vi "Autonomous Independent.vi"   [LabVIEW 2014]
doc: "This VI is called when autonomous begins, and will automatically be terminated when autonomous ends. You can carry out timed or sensor driven robot movement independently without needing to return to the caller."
uses:
  <vilib>/Rock Robotics/WPI/Joystick/WPI_JoystickGetSetRefNum.vi
  <vilib>/Rock Robotics/Network Tables/SD Write Numeric Array.vi
  Robot Global Data.vi
  <vilib>/Rock Robotics/WPI/RobotDrive/WPI_RobotDriveGetSetRefNum.vi
types:
  T1 = typedef "WPI_JoystickDevRef.ctl" = cluster{"Device":T2}
  T2 = typedef "WPI_JoystickDeviceEnum.ctl" = enum16{"USB 0", "USB 1", "USB 2", "USB 3", "USB 4", "USB 5"}
  T3 = typedef "WPI_RobotDriveDevRef.ctl" = cluster{"DevStatus":errorcluster, "Motors[]":T4[], "Square Inputs":bool, "Max Output":dbl}
  T4 = typedef "WPI_MotorControlDeviceRef.ctl" = cluster{"DeviceStatus":errorcluster, "Type":T5, "PWM":cluster{"Controller":T6, "PWM Channel":T7, "DeadBand":T8}, "CAN":cluster{"Device Number":u8, "Control Mode":T9, "Semaphore":T10, "Max Vout":dbl, "TalonSRX Control Mode":T11}, "Invert":bool, "TransformRef":T12, "InvTransformRef":T12}
  T5 = typedef "WPI_MotorControlType.ctl" = enum16{"PWM", "CAN", "CANTalonSRX"}
  T6 = typedef "FPGA_TypedefDigitalModule.ctl" = enum16{"Controller 1"}
  T7 = typedef "FPGA_DIOPWMChannel.ctl" = enum8{"PWM 0", "PWM 1", "PWM 2", "PWM 3", "PWM 4", "PWM 5", "PWM 6", "PWM 7", "PWM 8", "PWM 9", "PWM MXP 0", "PWM MXP 1", "PWM MXP 2", "PWM MXP 3", "PWM MXP 4", "PWM MXP 5", "PWM MXP 6", "PWM MXP 7", "PWM MXP 8", "PWM MXP 9", "Invalid"}
  T8 = typedef "WPI_PWMDeadband.ctl" = cluster{"Name":string, "maxPositivePwm":i32, "minPositivePwm":i32, "centerPwm":i32, "maxNegativePwm":i32, "minNegativePwm":i32, "angularRange":u16}
  T9 = typedef "WPI_CANJaguar_ControlMode.ctl" = enum8{"Percent VBus", "Current", "Speed", "Position", "Voltage"}
  T10 = typedef "Semaphore RefNum" = refnum<k1>
  T11 = typedef "WPI_CANTalonSRX_APIControlMode.ctl" = enum8{"Percent VBus", "Speed", "Position", "Slave", "Unchanged / Invalid"}
  T12 = typedef "WPI_PWMTransform_ConPane.ctl" = refnum<vi>
  T13 = typedef "WPI_CANTalonSRX_GlobalStatus.ctl" = cluster{"Applied Throttle":dbl, "Module Enabled":bool, "CAN Error":errorcluster, "Closed Loop Error":dbl, "Forward Limit Switch Closed":bool, "Reverse Limit Switch Closed":bool, "Sensor Position":dbl, "Sensor Velocity":dbl, "Current":dbl, "Sticky Fault - Over Temp":bool, "Sticky Fault - Under Voltage":bool, "Sticky Fault - Forward Limit":bool, "Sticky Fault - Reverse Limit":bool, "Sticky Fault - Forward Soft Limit":bool, "Sticky Fault - Reverse Soft Limit":bool, "Brake is Enabled":bool, "Encoder Position":dbl, "Encoder Velocity":dbl, "Encoder Index Count":dbl, "Encoder A Pin State":bool, "Encoder B Pin State":bool, "Encoder Index Pin State":bool, "Analog In":dbl, "Analog In Velocity":dbl, "Temperature (C)":dbl, "Battery Voltage":dbl}
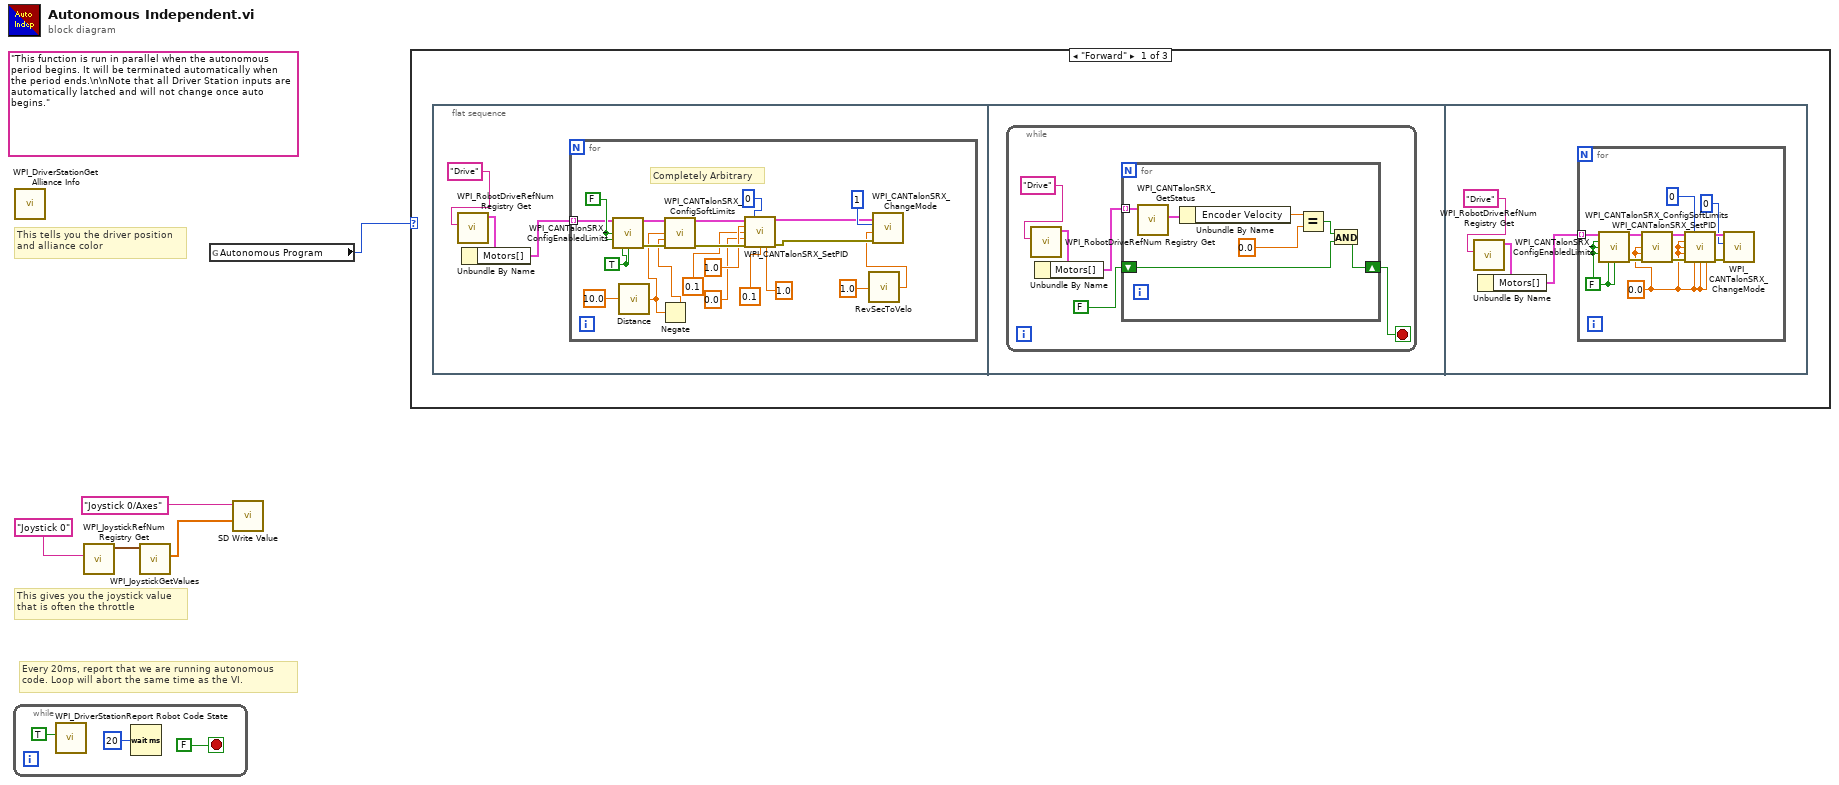
[diagram p0: block diagram]
diagram:
  (unwired) "This function is run in parallel when the autonomous period begins. It will be terminated automatically when the period ends.\n\nNote that all Driver Station inputs are automatically latched and will not change once auto begins."
  # "Every 20ms, report that we are running autonomous\ncode. Loop will abort the same time as the VI."
  # "This gives you the joystick value\nthat is often the throttle"
  # "This tells you the driver position\nand alliance color"
  n1 = while {
    stop <- FALSE stop-if-true
    n2 = call <vilib>:"WPI_DriverStationReport Robot Code State.vi"("Autonomous"=TRUE) -> ()  [unwired: 10 in, 1 out]
    n3 = Wait (ms)(milliseconds to wait=u32 20) -> ()  [unwired: 1 out]
  }
  n4 = call <vilib>:"WPI_DriverStationGet Alliance Info.vi"() -> ()  [unwired: 12 out]
  n5 = call <vilib>:"WPI_JoystickRefNum Registry Get.vi"("refnum name"="Joystick 0") -> ("JoystickDevRef"=w4:T1)  [unwired: 1 in, 9 out]
  n6 = call <vilib>:"WPI_JoystickGetValues.vi"("JoystickDevRef"=w4) -> ("Axes"=w2:dbl[])  [unwired: 6 in, 4 out]
  n7 = global read "Robot Global Data.vi" "Autonomous Program"() -> (w1:enum16{"Forward", "Stack", "Null"})
  n8 = call-poly <vilib>:"SD Write Value.vi"("Numeric Array"=w2, "Name"="Joystick 0/Axes") -> ()  [unwired: 8 in, 2 out]
  n9 = case shown="\"Forward\"" w1 {
    frame "Forward" {
      n10 = flat-sequence {
        frame #0 {
          n11 = call <vilib>:"WPI_RobotDriveRefNum Registry Get.vi"("refnum name"="Drive") -> ("RobotDriveDevRef"=w11:T3)  [unwired: 9 in, 1 out]
          n12 = Unbundle By Name(w11) -> ("Motors[]"=w9:T4[])
          n13 = for {
            tunnel: w9 -> [w17] mode=indexing
            w31 = TRUE
            w32 = FALSE
            # "Completely Arbitrary"
            n14 = call <vilib>:"WPI_CANTalonSRX_ConfigEnabledLimits.vi"("CAN Talon SRX Ref"=w17, "Forward Limit Switch Enable"=w32, "Reverse Limit Switch Enable"=w32, "Forward Soft Limit Enable"=w31, "Reverse Soft Limit Enable"=w31) -> ("CAN Talon SRX Ref Out"=w30:T4, "error out"=w29:errorcluster)  [unwired: 9 in]
            n15 = call "Distance.vi"("Revolutions"=10.0) -> ("Distance"=w13:dbl)
            n16 = Negate(x=w13) -> (-x=w12:dbl)
            n17 = call <vilib>:"WPI_CANTalonSRX_ConfigSoftLimits.vi"("CAN Talon SRX Ref"=w30, "Forward Limit Position"=w13, "Reverse Limit Position"=w12, "error in (no error)"=w29) -> ("CAN Talon SRX Ref Out"=w27:T4, "error out"=w26:errorcluster)  [unwired: 10 in]
            n18 = call <vilib>:"WPI_CANTalonSRX_SetPID.vi"("CAN Talon SRX Ref"=w27, "Parameter Slot"=0, "P"=1.0, "I"=0.1, "D"=0.0, "error in (no error)"=w26, "I Zone"=0.1, "Ramp Rate"=1.0) -> ("CAN Talon SRX Ref Out"=w24:T4, "error out"=w25:errorcluster)  [unwired: 6 in]
            n19 = call "RevSecToVelo.vi"("Revolutions/s"=1.0) -> ("Velocity"=w15:dbl)
            n20 = call <vilib>:"WPI_CANTalonSRX_ChangeMode.vi"("error in (no error)"=w25, "Output"=w15, "Control Mode"=1, "CAN Talon SRX Ref"=w24) -> ()  [unwired: 6 in, 2 out]
          }
        }
        frame #1 {
          n21 = while {
            stop <- w33 stop-if-true
            n22 = call <vilib>:"WPI_RobotDriveRefNum Registry Get.vi"("refnum name"="Drive") -> ("RobotDriveDevRef"=w36:T3)  [unwired: 9 in, 1 out]
            n23 = Unbundle By Name(w36) -> ("Motors[]"=w35:T4[])
            n24 = for {
              tunnel: w35 -> [w41] mode=indexing
              shift-right: [w39] -> w33
              shift-left: FALSE -> [w38]
              n25 = call <vilib>:"WPI_CANTalonSRX_GetStatus.vi"("CAN Talon SRX Ref"=w41) -> ("Talon SRX Status"=w44:T13)  [unwired: 8 in, 2 out]
              n26 = Unbundle By Name(w44) -> ("Encoder Velocity"=w43:dbl)
              n27 = Equal?(x=w43, y=0.0) -> (x = y?=w40:bool)
              n28 = And(x=w40, y=w38) -> (x .and. y?=w39:bool)
            }
          }
        }
        frame #2 {
          n29 = call <vilib>:"WPI_RobotDriveRefNum Registry Get.vi"("refnum name"="Drive") -> ("RobotDriveDevRef"=w46:T3)  [unwired: 9 in, 1 out]
          n30 = Unbundle By Name(w46) -> ("Motors[]"=w45:T4[])
          n31 = for {
            tunnel: w45 -> [w58] mode=indexing
            w51 = 0.0
            w57 = FALSE
            n32 = call <vilib>:"WPI_CANTalonSRX_ConfigEnabledLimits.vi"("CAN Talon SRX Ref"=w58, "Override Limit Switches"=w57, "Forward Limit Switch Enable"=w57, "Reverse Limit Switch Enable"=w57, "Forward Soft Limit Enable"=w57, "Reverse Soft Limit Enable"=w57) -> ("CAN Talon SRX Ref Out"=w56:T4, "error out"=w55:errorcluster)  [unwired: 8 in]
            n33 = call <vilib>:"WPI_CANTalonSRX_ConfigSoftLimits.vi"("CAN Talon SRX Ref"=w56, "Forward Limit Position"=w51, "Reverse Limit Position"=w51, "error in (no error)"=w55) -> ("CAN Talon SRX Ref Out"=w54:T4, "error out"=w53:errorcluster)  [unwired: 10 in]
            n34 = call <vilib>:"WPI_CANTalonSRX_SetPID.vi"("CAN Talon SRX Ref"=w54, "Parameter Slot"=0, "P"=w51, "I"=w51, "D"=w51, "error in (no error)"=w53, "F"=w51, "I Zone"=w51, "Ramp Rate"=w51) -> ("CAN Talon SRX Ref Out"=w49:T4, "error out"=w50:errorcluster)  [unwired: 5 in]
            n35 = call <vilib>:"WPI_CANTalonSRX_ChangeMode.vi"("error in (no error)"=w50, "Control Mode"=0, "CAN Talon SRX Ref"=w49) -> ()  [unwired: 7 in, 2 out]
          }
        }
      }
    }
    frame "Stack" {
    }
    frame "Null", Default {
    }
  }
